vi "UDP Tx Process.vi"(10 "Parameters":variant, 11 "Process":refnum<class "Process.lvclass">) -> ()   [LabVIEW 2019, in "UDP-Custom-Device Engine.lvlib"]
uses:
  UDP-Custom-Device Engine.lvlib
  <vilib>/NI/NIVS Inline Async API/_VS Inline Async API/Process/Process.lvclass
  <vilib>/NI/NIVS Inline Async API/_VS Inline Async API/Process/Process.lvclass/Process.ctl
  <vilib>/NI/NIVS Inline Async API/_VS Inline Async API/Process/Data Member Access/Read Data Access.vi
  <vilib>/NI/NIVS Inline Async API/_VS Inline Async API/Error Handling Process/SubVIs/Error.ConvertArray.vi
  <vilib>/NI/NIVS Inline Async API/_Data Access Engine/Data Access Engine/Data Access Engine.lvclass
  <vilib>/NI VeriStand/VeriStand Data/VeriStand Data.lvlib
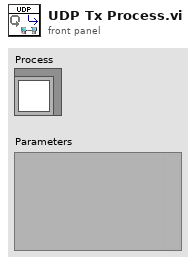
[diagram p1: front panel]
types:
  T1 = typedef "UDP-Custom-Device Engine.lvlib/Engine - Tx Loop Data.ctl" = cluster{"General Resources":T2, "Header Details":T4, "Data Conversion":T5, "Runtime Resources":T7, "Echo Resources":T11, "Channel Resources":T13, "Debug Resources":T16}
  T2 = typedef "UDP-Custom-Device Engine.lvlib/Engine - General Resources.ctl" = cluster{"Packet Name":string, "Packet ID":i32, "Local IP Address":string, "Local Port":i32, "Multicast":bool, "Multicast IP Address":u32, "Header Info":bool[], "Byte Order":enum16{"big-endian, network order", "native, host order", "little-endian"}, "Channel Data Types":T3[], "Duplex Packets":refnum<data-value>}
  T3 = typedef "VeriStand Data.lvlib/Typedefs.Data Types.ctl" = enum16{"Boolean", "Single", "Double", "I8", "I16", "I32", "I64", "U8", "U16", "U32", "U64"}
  T4 = typedef "UDP-Custom-Device Shared.lvlib/Shared - Header Details.ctl" = cluster{"Packet Size":u16, "Protocol Revision":u8, "System Definition Version":u64, "Source Node Name":string, "Packet ID":u32, "Number of Channels":u32, "Static Header Size":u16, "Total Header Size":u16}
  T5 = typedef "UDP-Custom-Device Engine.lvlib/Engine - Data Conversion Config.ctl" = cluster{"Byte Buffer":refnum<class "Byte Buffer.lvclass">, "Data Pointers":u64[], "Channel Count":i32, "Mappings":T6[], "Static Header Payload":string, "Packet Count":dbl, "Packet Size":i32}
  T6 = typedef "VeriStand Data.lvlib/Byte Buffer.lvclass/Byte Buffer.Mapping.ctl" = cluster{"pointer":u64, "count":i64, "buffer offset":u64, "data type":T3}
  T7 = typedef "UDP-Custom-Device Engine.lvlib/Engine - Tx Runtime Resources.ctl" = cluster{"Connection ID":refnum<k16>, "Transmit Option":T8, "Destination IP Address":u32, "Destination Port":u16, "Multicast IP Address":u32, "TTL":u16, "Multicast":bool, "Port as Channel":bool, "ExecutionConfig":T9}
  T8 = typedef "UDP-Custom-Device Shared.lvlib/Shared - Transmit Flag Options.ctl" = enum16{"Always", "One-Shot", "Toggle"}
  T9 = typedef "UDP-Custom-Device Engine.lvlib/Engine - Execution Config.ctl" = cluster{"Loop Period":i64, "RT Loop Period":i64, "Untimed Period":u32, "Target Processor":i32, "Priority":i32, "Thread Management":T10}
  T10 = typedef "UDP-Custom-Device Shared.lvlib/Shared - Thread Management.ctl" = enum16{"Untimed (Default)", "Timed (High Priority)"}
  T11 = typedef "UDP-Custom-Device Engine.lvlib/Engine - Tx Echo Resources.ctl" = cluster{"Transmit Echo Option":T12, "Packet Count":dbl, "Counter Increment":dbl, "Transmit Values":dbl[]}
  T12 = typedef "UDP-Custom-Device Shared.lvlib/Shared - Transmit Echo Options.ctl" = enum16{"PCL Reset", "Counter", "Mirror"}
  T13 = typedef "UDP-Custom-Device Engine.lvlib/Engine - Tx Channel Refs.ctl" = cluster{"Transmit Channels":T14, "Transmit Flag":T14, "Transmit Echo":T15, "Port Channel":T14}
  T14 = typedef "Data Access Engine.lvlib/Data Access Engine.lvclass/Read.DVR.ctl" = refnum<data-value>
  T15 = typedef "Data Access Engine.lvlib/Data Access Engine.lvclass/Write.DVR.ctl" = refnum<data-value>
  T16 = typedef "UDP-Custom-Device Engine.lvlib/Engine - Debug Resources.ctl" = cluster{"Debug Mode":bool, "Debug Log File":refnum<file>, "Packet Name":string}
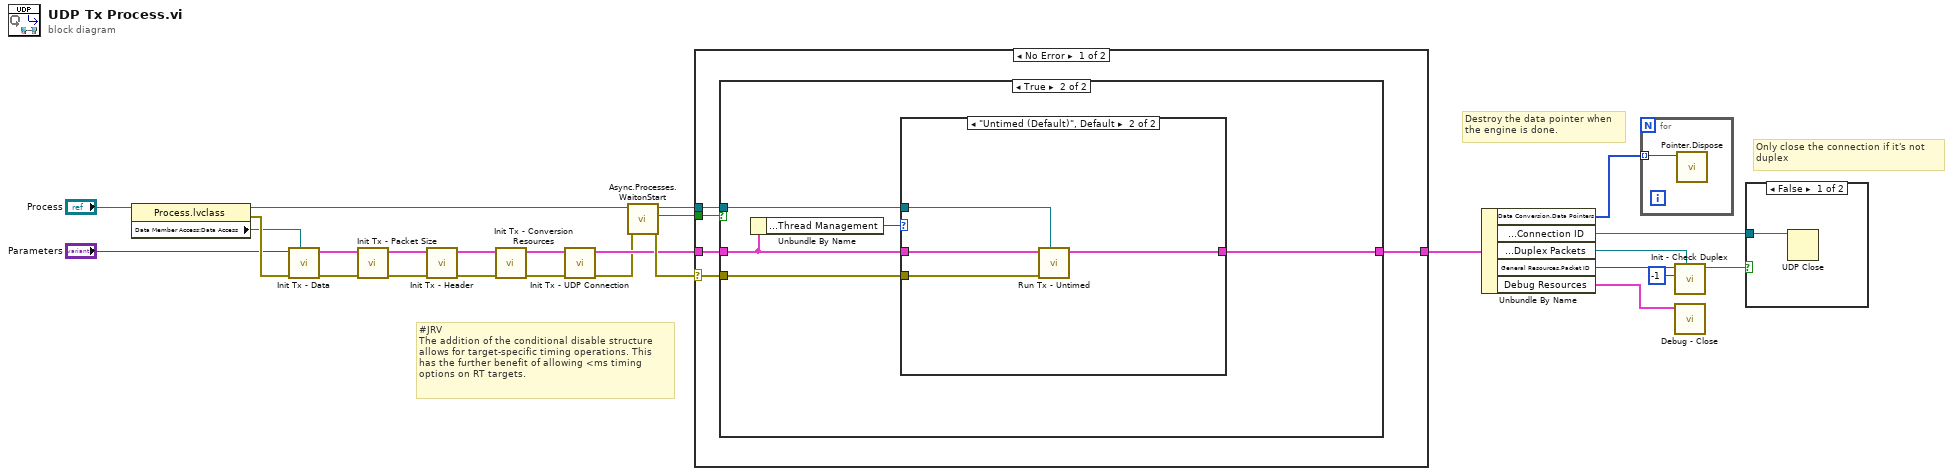
[diagram p0: block diagram]
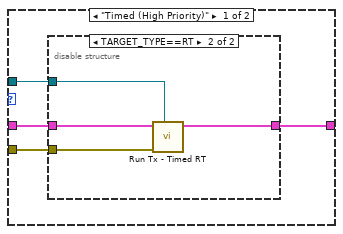
[diagram p3: hidden frame]
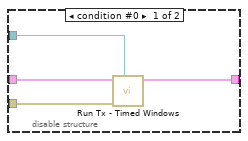
[diagram p4: hidden frame]
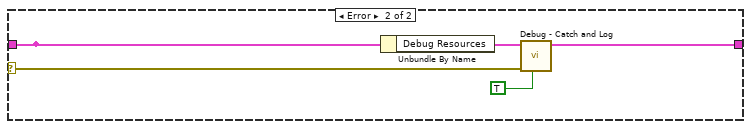
[diagram p5: hidden frame]
diagram:
  # "#JRV\nThe addition of the conditional disable structure\nallows for target-specific timing operations. This\nhas the further benefit of allowing <ms timing\noptions on RT targets."
  # "Only close the connection if it's not\nduplex"
  # "Destroy the data pointer when\nthe engine is done."
  n1 = property class="Process.lvclass"(reference="Process") -> (reference out=w26:refnum<class "Process.lvclass">, error out=w21:errorcluster, "Data Member Access:Data Access"=w17:refnum<class "Data Access Engine.lvclass">)  [unwired: 1 in]
  n2 = call "Init Tx - Data.vi"("Data Access in"=w17, "error in (no error)"=w21, "Parameters"="Parameters") -> ("error out"=w9:errorcluster, "Tx Loop Data"=w6:T1)  [unwired: 6 in, 1 out]
  n3 = call "Init Tx - Packet Size.vi"("error in (no error)"=w9, "Tx Loop Data"=w6) -> ("error out"=w8:errorcluster, "Tx Loop Data out"=w10:T1)  [unwired: 8 in]
  n4 = call "Init Tx - Header.vi"("error in (no error)"=w8, "Tx Loop Data"=w10) -> ("error out"=w11:errorcluster, "Tx Loop Data out"=w12:T1)  [unwired: 8 in]
  n5 = call "Init Tx - Conversion Resources.vi"("error in (no error)"=w11, "Tx Loop Data"=w12) -> ("error out"=w15:errorcluster, "Tx Loop Data out"=w16:T1)  [unwired: 8 in]
  n6 = call "Init Tx - UDP Connection.vi"("error in (no error)"=w15, "Tx Loop Data in"=w16) -> ("error out"=w18:errorcluster, "Tx Loop Data out"=w19:T1)  [unwired: 8 in]
  n7 = call <vilib>:"Async.Processes.WaitonStart.vi"("error in (no error)"=w18, "Process"=w26) -> ("error out"=w24:errorcluster, "Execute"=w22:bool, "Process out"=w23:refnum<class "Process.lvclass">)  [unwired: 7 in]
  n8 = case shown="No Error" w24 {
    selector: w24 -> [w29 w55]
    tunnel: w22 -> [w31 _]
    tunnel: w23 -> [w30 _]
    tunnel: w19 -> [w28 w54]
    tunnel: [w27 w54] -> w13
    frame No Error {
      n9 = case shown="True" w31 {
        tunnel: w29 -> [_ w36]
        tunnel: w30 -> [_ w37]
        tunnel: w28 -> [w32 w34]
        tunnel: [w32 w35] -> w27
        frame False {
        }
        frame True {
          n10 = Unbundle By Name(w34) -> ("Runtime Resources.ExecutionConfig.Thread Management"=w33:T10)
          n11 = case shown="\"Untimed (Default)\", Default" w33 {
            tunnel: w37 -> [w41 w51]
            tunnel: w36 -> [w40 w52]
            tunnel: [w39 w50] -> w35
            tunnel: w34 -> [w38 w53]
            frame "Timed (High Priority)" {
              n12 = disable-structure shown="TARGET_TYPE==RT" {
                disable-tunnel: w41 -> [w44 w49]
                disable-tunnel: w40 -> [w43 w47]
                disable-tunnel: w38 -> [w45 w48]
                disable-tunnel: [w42 w46] -> w39
                frame condition #0 {
                  n13 = call "Run Tx - Timed Windows.vi"("Process in"=w44, "error in (no error)"=w43, "Tx Loop Data in"=w45) -> ("Tx Loop Data out"=w42:T1)  [unwired: 8 in]
                }
                frame condition #1 (active) {
                  n14 = call "Run Tx - Timed RT.vi"("Process in"=w49, "error in (no error)"=w47, "Tx Loop Data in"=w48) -> ("Tx Loop Data out"=w46:T1)  [unwired: 8 in]
                }
              }
            }
            frame "Untimed (Default)", Default {
              n15 = call "Run Tx - Untimed.vi"("Process in"=w51, "error in (no error)"=w52, "Tx Loop Data in"=w53) -> ("Tx Loop Data out"=w50:T1)  [unwired: 8 in]
            }
          }
        }
      }
    }
    frame Error {
      n16 = Unbundle By Name(w54) -> ("Debug Resources"=w56:T16)
      n17 = call "Debug - Catch and Log.vi"("Clear Error?"=TRUE, "error in (no error)"=w55, "Debug Resources"=w56) -> ()  [unwired: 8 in, 1 out]
    }
  }
  n18 = Unbundle By Name(w13) -> ("Data Conversion.Data Pointers"=w14:u64[], "Runtime Resources.Connection ID"=w7:refnum<k16>, "General Resources.Duplex Packets"=w5:refnum<data-value>, "General Resources.Packet ID"=w4:i32, "Debug Resources"=w1:T16)
  n19 = for {
    tunnel: w14 -> [w58] mode=indexing
    n20 = call <vilib>:"Pointer.Dispose.vi"("pointer"=w58) -> ()  [unwired: 9 in, 2 out]
  }
  n21 = call "Init - Check Duplex.vi"("Duplex Packets"=w5, "Receive Packet ID"=-1, "Transmit Packet ID"=w4) -> ("Is Duplex?"=w2:bool)  [unwired: 6 in, 2 out]
  n22 = call "Debug - Close.vi"("Debug Resources"=w1) -> ()  [unwired: 10 in, 1 out]
  n23 = case shown="False" w2 {
    tunnel: w7 -> [w59 _]
    frame False {
      n24 = UDP Close(connection ID=w59) -> ()  [unwired: 1 in, 2 out]
    }
    frame True {
    }
  }
